vi "Export Image.vi"(0 "Image Folder":path, 2 "Filename":string, 3 "Type":string, 8 "File Directory":path) -> ()   [LabVIEW 2017, in "DocTools.lvlib"]
uses:
  DocTools.lvlib
panel:
  out "String":string
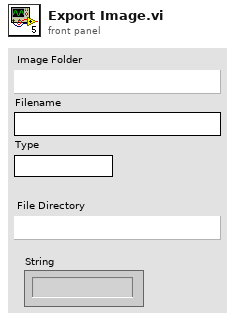
[diagram p1: front panel]
types:
  T1 = typedef "imagedata.ctl" = cluster{"image type":i32, "image depth":i32, "image":u8[], "mask":u8[], "colors":u32[], "Rectangle":cluster{"left":i16, "top":i16, "right":i16, "bottom":i16}}
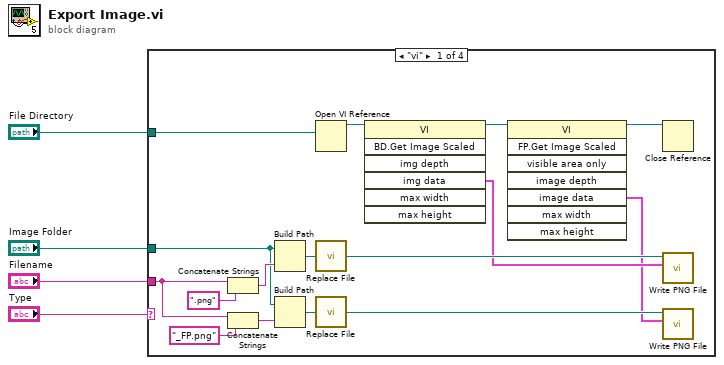
[diagram p0: block diagram]
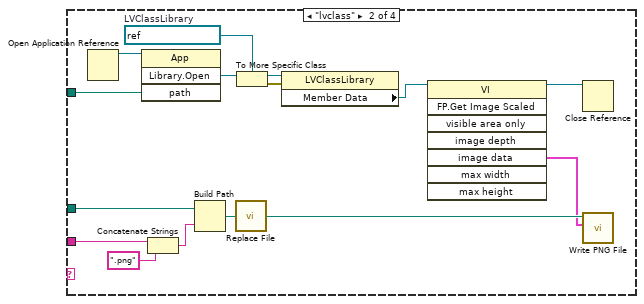
[diagram p2: hidden frame]
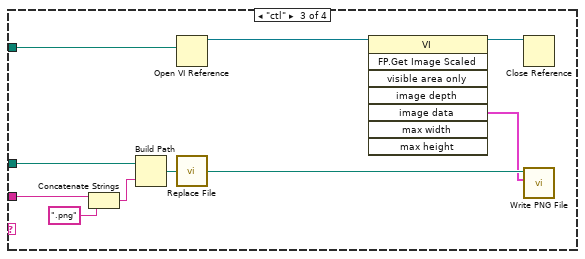
[diagram p3: hidden frame]
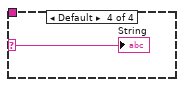
[diagram p4: hidden frame]
diagram:
  n1 = case shown="\"vi\"" "Type" {
    selector: "Type" -> [_ _ _ w46]
    tunnel: "Filename" -> [w18 w34 w44 _]
    tunnel: "Image Folder" -> [w16 w32 w42 _]
    tunnel: "File Directory" -> [w12 w26 w40 _]
    frame "vi" {
      n2 = Concatenate Strings(w18, ".png" ("string")) -> (w17:string)
      n3 = Concatenate Strings(w18, "_FP.png" ("string")) -> (w15:string)
      n4 = Build Path(base path=w16, name or relative path=w17) -> (appended path=w14:path)
      n5 = Build Path(base path=w16, name or relative path=w15) -> (appended path=w13:path)
      n6 = Open VI Reference(vi path=w12) -> (vi reference=w11:refnum<vi>)  [unwired: 5 in, 1 out]
      n7 = call "Replace File.vi"("File In"=w14) -> ("File Out"=w8:path)
      n8 = call "Replace File.vi"("File In"=w13) -> ("File Out"=w6:path)
      n9 = invoke class="VI" method="BD.Get Image Scaled"(reference=w11) -> (reference out=w10:refnum<vi>, "img data"=w7:T1)  [unwired: 6 in, 5 out]
      n10 = invoke class="VI" method="FP.Get Image Scaled"(reference=w10) -> (reference out=w9:refnum<vi>, "image data"=w5:T1)  [unwired: 7 in, 6 out]
      n11 = Close Reference(reference=w9) -> ()  [unwired: 1 in, 1 out]
      n12 = call <vilib>:"Write PNG File.vi"("image data"=w7, "path to PNG file"=w8) -> ()  [unwired: 8 in, 2 out]
      n13 = call <vilib>:"Write PNG File.vi"("image data"=w5, "path to PNG file"=w6) -> ()  [unwired: 8 in, 2 out]
    }
    frame "lvclass" {
      w24 = refnum<vi> refnum  # LVClassLibrary
      n14 = Open Application Reference() -> (3:w27:refnum<vi>)  [unwired: 4 in, 1 out]
      n15 = invoke class="App" method="Library.Open"(reference=w27, "path"=w26) -> ("Open Library"=w25:refnum<vi>)  [unwired: 2 in, 3 out]
      n16 = Concatenate Strings(w34, ".png" ("string")) -> (w33:string)
      n17 = Build Path(base path=w32, name or relative path=w33) -> (appended path=w31:path)
      n18 = call "Replace File.vi"("File In"=w31) -> ("File Out"=w29:path)
      n19 = To More Specific Class(target class=w24, reference=w25) -> (specific class reference=w23:refnum<vi>, error out=w22:errorcluster)  [unwired: 1 in]
      n20 = property class="LVClassLibrary"(reference=w23, error in=w22) -> ("Member Data"=w21:refnum<vi>)  [unwired: 2 out]
      n21 = invoke class="VI" method="FP.Get Image Scaled"(reference=w21) -> (reference out=w30:refnum<vi>, "image data"=w28:T1)  [unwired: 7 in, 6 out]
      n22 = Close Reference(reference=w30) -> ()  [unwired: 1 in, 1 out]
      n23 = call <vilib>:"Write PNG File.vi"("image data"=w28, "path to PNG file"=w29) -> ()  [unwired: 8 in, 2 out]
    }
    frame "ctl" {
      n24 = Concatenate Strings(w44, ".png" ("string")) -> (w43:string)
      n25 = Build Path(base path=w42, name or relative path=w43) -> (appended path=w41:path)
      n26 = Open VI Reference(vi path=w40) -> (vi reference=w39:refnum<vi>)  [unwired: 5 in, 1 out]
      n27 = call "Replace File.vi"("File In"=w41) -> ("File Out"=w37:path)
      n28 = invoke class="VI" method="FP.Get Image Scaled"(reference=w39) -> (reference out=w38:refnum<vi>, "image data"=w36:T1)  [unwired: 7 in, 6 out]
      n29 = Close Reference(reference=w38) -> ()  [unwired: 1 in, 1 out]
      n30 = call <vilib>:"Write PNG File.vi"("image data"=w36, "path to PNG file"=w37) -> ()  [unwired: 8 in, 2 out]
    }
    frame Default {
      "String" <- w46
    }
  }
